vi "Disabled.vi"(7 "Robot Mode":T2, 10 "Match Info":T1={"Autonomous Elapsed Seconds"=0.0, "TeleOp Elapsed Seconds"=0.0, "Disabled Elapsed Seconds"=0.0, "Visited Autonomous"=FALSE, "Visited TeleOp"=FALSE, "Visited Disabled"=FALSE, "Autonomous Settings"={"Autonomous Style"=enum."Independent", "VI Refnum"=refnum}}, 11 "Call Context":T3) -> ()   [LabVIEW 2012]
doc: "This VI is called each time a disabled packet is received from the DS. It is often used to prepare for the next robot mode, to calibrate sensors, etc."
uses:
  <vilib>/Rock Robotics/WPI/DriverStation/WPI_DriverStationDerivedRobotMode.ctl
  <vilib>/Rock Robotics/WPI/DriverStation/WPI_DriverStationRobotMode2.ctl
  <vilib>/Rock Robotics/WPI/DriverStation/WPI_DriverStationMatch Info.ctl
  Robot Global Data.vi
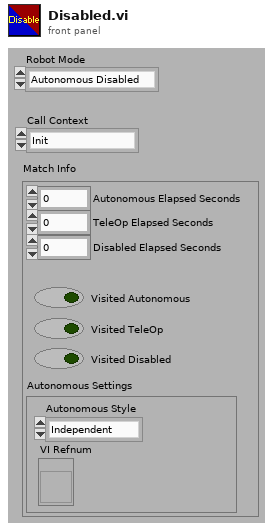
[diagram p1: front panel]
types:
  T1 = typedef "WPI_DriverStationMatch Info.ctl" = cluster{"Autonomous Elapsed Seconds":dbl, "TeleOp Elapsed Seconds":dbl, "Disabled Elapsed Seconds":dbl, "Visited Autonomous":bool, "Visited TeleOp":bool, "Visited Disabled":bool, "Autonomous Settings":cluster{"Autonomous Style":enum16{"Iterative", "Independent"}, "VI Refnum":refnum<vi>}}
  T2 = typedef "WPI_DriverStationRobotMode2.ctl" = enum16{"Autonomous Disabled", "Autonomous Enabled", "Teleop Disabled", "Teleop Enabled", "Timeout", "Finish", "Test Disabled", "Test Enabled"}
  T3 = typedef "WPI_DriverStationDerivedRobotMode.ctl" = enum16{"Init", "Execute", "Stop"}
  T4 = cluster{"FlipperLeftUp":dbl, "FlipperLeftDown":dbl, "FlipperRightUp":dbl, "FlipperRightDown":dbl, "KickerLeftBack":dbl, "KickerLeftForward":dbl, "KickerRightBack":dbl, "KickerRightForward":dbl}
  T5 = typedef "WPI_MotorControlDeviceRef.ctl" = cluster{"DeviceStatus":errorcluster, "Type":enum16{"PWM", "CAN"}, "PWM":cluster{"Digital Module":T6, "PWM Channel":T7, "DeadBand":T8}, "CAN":cluster{"Device Number":u8, "Control Mode":T9, "Semaphore":T10, "Max Vout":dbl}, "Invert":bool, "TransformRef":T11, "InvTransformRef":T11}
  T6 = typedef "FPGA_TypedefDigitalModule.ctl" = enum16{"Digital Module 1", "Digital Module 2"}
  T7 = typedef "FPGA_DIOPWMChannel.ctl" = enum8{"PWM 1", "PWM 2", "PWM 3", "PWM 4", "PWM 5", "PWM 6", "PWM 7", "PWM 8", "PWM 9", "PWM 10", "Invalid"}
  T8 = typedef "WPI_PWMDeadband.ctl" = cluster{"Name":string, "maxPositivePwm":i32, "minPositivePwm":i32, "centerPwm":i32, "maxNegativePwm":i32, "minNegativePwm":i32, "angularRange":u16}
  T9 = typedef "WPI_CANJaguar_ControlMode.ctl" = enum8{"Percent VBus", "Current", "Speed", "Position", "Voltage"}
  T10 = typedef "Semaphore RefNum" = refnum<k1>
  T11 = typedef "WPI_PWMTransform_ConPane.ctl" = refnum<vi>
  T12 = typedef "WPI_ServoDeviceRef.ctl" = cluster{"DeviceStatus":errorcluster, "Digital Module":T6, "PWM Channel":T7, "DeadBand":T8}
  T13 = cluster{"Right Servo High":dbl, "Right Servo Mid":dbl, "Right Servo Low":dbl, "Left Servo High":dbl, "Left Servo Mid":dbl, "Left Servo Low":dbl}
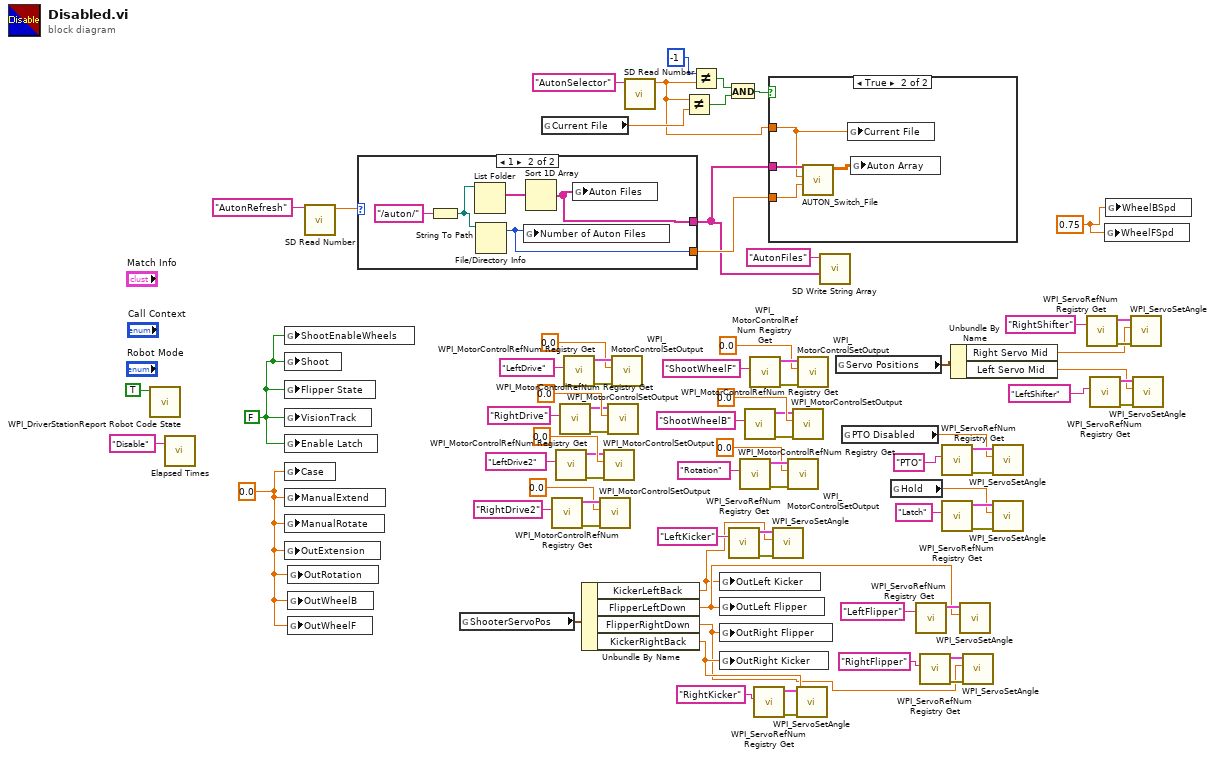
[diagram p0: block diagram]
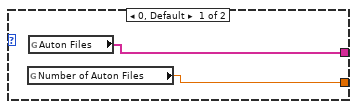
[diagram p3: hidden frame]
diagram:
  w1 = 0.75 ("Case")
  w24 = 0.0 ("Case")
  w25 = FALSE ("Enable Latch")
  n1 = call <vilib>:"WPI_DriverStationReport Robot Code State.vi"("Disabled"=TRUE ("Autonomous")) -> ()  [unwired: 10 in, 1 out]
  n2 = call "Elapsed Times.vi"("Call Name"="Disable") -> ()  [unwired: 2 in, 1 out]
  n3 = global write "Robot Global Data.vi" "ShootEnableWheels"(w25) -> ()
  n4 = global write "Robot Global Data.vi" "Shoot"(w25) -> ()
  n5 = global write "Robot Global Data.vi" "Flipper State"(w25) -> ()
  n6 = global write "Robot Global Data.vi" "VisionTrack"(w25) -> ()
  n7 = global write "Robot Global Data.vi" "Enable Latch"(w25) -> ()
  n8 = global write "Robot Global Data.vi" "Case"(w24) -> ()
  n9 = global write "Robot Global Data.vi" "ManualExtend"(w24) -> ()
  n10 = global write "Robot Global Data.vi" "ManualRotate"(w24) -> ()
  n11 = global write "Robot Global Data.vi" "OutExtension"(w24) -> ()
  n12 = global write "Robot Global Data.vi" "OutRotation"(w24) -> ()
  n13 = global write "Robot Global Data.vi" "OutWheelB"(w24) -> ()
  n14 = global write "Robot Global Data.vi" "OutWheelF"(w24) -> ()
  n15 = call <vilib>:"SD Read Number.vi"("Name"="AutonRefresh") -> ("Numeric"=w58:dbl)  [unwired: 8 in, 2 out]
  n16 = case shown="1" w58 {
    tunnel: [w79 w82] -> w68
    tunnel: [w80 w81] -> w63
    frame 0, Default {
      n17 = global read "Robot Global Data.vi" "Number of Auton Files"() -> (w79:dbl)
      n18 = global read "Robot Global Data.vi" "Auton Files"() -> (w80:string[])
    }
    frame 1 {
      n19 = String To Path(string="/auton/") -> (path=w84:path)
      n20 = List Folder(path=w84) -> (filenames=w83:string[])  [unwired: 3 in, 3 out]
      n21 = File/Directory Info(path=w84) -> (size=w82:i64)  [unwired: 1 in, 6 out]
      n22 = global write "Robot Global Data.vi" "Number of Auton Files"(w82) -> ()
      n23 = Sort 1D Array(array=w83) -> (sorted array=w81:string[])
      n24 = global write "Robot Global Data.vi" "Auton Files"(w81) -> ()
    }
  }
  n25 = global read "Robot Global Data.vi" "ShooterServoPos"() -> (w23:T4)
  n26 = global read "Robot Global Data.vi" "Current File"() -> (w66:dbl)
  n27 = call <vilib>:"WPI_MotorControlRefNum Registry Get.vi"("refnum name"="RightDrive2") -> ("error out"=w44:errorcluster, "MotorControlDevRef"=w43:T5)  [unwired: 9 in]
  n28 = call <vilib>:"WPI_MotorControlRefNum Registry Get.vi"("refnum name"="LeftDrive2") -> ("error out"=w37:errorcluster, "MotorControlDevRef"=w38:T5)  [unwired: 9 in]
  n29 = call <vilib>:"WPI_MotorControlRefNum Registry Get.vi"("refnum name"="RightDrive") -> ("error out"=w69:errorcluster, "MotorControlDevRef"=w70:T5)  [unwired: 9 in]
  n30 = call <vilib>:"WPI_MotorControlRefNum Registry Get.vi"("refnum name"="LeftDrive") -> ("error out"=w76:errorcluster, "MotorControlDevRef"=w75:T5)  [unwired: 9 in]
  n31 = Unbundle By Name(w23) -> ("KickerLeftBack"=w20:dbl, "FlipperLeftDown"=w21:dbl, "FlipperRightDown"=w19:dbl, "KickerRightBack"=w22:dbl)
  n32 = call <vilib>:"WPI_MotorControlSetOutput.vi"("error in (no error)"=w44, "Output"=0.0, "MotorControlDevRef"=w43) -> ()  [unwired: 6 in, 3 out]
  n33 = call <vilib>:"WPI_MotorControlSetOutput.vi"("error in (no error)"=w37, "Output"=0.0, "MotorControlDevRef"=w38) -> ()  [unwired: 6 in, 3 out]
  n34 = call <vilib>:"WPI_MotorControlSetOutput.vi"("error in (no error)"=w69, "Output"=0.0, "MotorControlDevRef"=w70) -> ()  [unwired: 6 in, 3 out]
  n35 = call <vilib>:"WPI_MotorControlSetOutput.vi"("error in (no error)"=w76, "Output"=0.0, "MotorControlDevRef"=w75) -> ()  [unwired: 6 in, 3 out]
  n36 = call <vilib>:"SD Read Number.vi"("Name"="AutonSelector") -> ("Numeric"=w59:dbl)  [unwired: 8 in, 2 out]
  n37 = Not Equal?(x=w59, y=w66) -> (x != y?=w64:bool)
  n38 = Not Equal?(x=-1, y=w59) -> (x != y?=w65:bool)
  n39 = global write "Robot Global Data.vi" "OutLeft Kicker"(w20) -> ()
  n40 = global write "Robot Global Data.vi" "OutLeft Flipper"(w21) -> ()
  n41 = global write "Robot Global Data.vi" "OutRight Flipper"(w19) -> ()
  n42 = global write "Robot Global Data.vi" "OutRight Kicker"(w22) -> ()
  n43 = And(x=w65, y=w64) -> (x .and. y?=w61:bool)
  n44 = call <vilib>:"WPI_ServoRefNum Registry Get.vi"("refnum name"="LeftKicker") -> ("error out"=w26:errorcluster, "ServoDeviceRef"=w27:T12)  [unwired: 9 in]
  n45 = call <vilib>:"WPI_MotorControlRefNum Registry Get.vi"("refnum name"="Rotation") -> ("error out"=w48:errorcluster, "MotorControlDevRef"=w47:T5)  [unwired: 9 in]
  n46 = call <vilib>:"WPI_MotorControlRefNum Registry Get.vi"("refnum name"="ShootWheelB") -> ("error out"=w49:errorcluster, "MotorControlDevRef"=w50:T5)  [unwired: 9 in]
  n47 = call <vilib>:"WPI_MotorControlRefNum Registry Get.vi"("refnum name"="ShootWheelF") -> ("error out"=w56:errorcluster, "MotorControlDevRef"=w55:T5)  [unwired: 9 in]
  n48 = call <vilib>:"WPI_ServoRefNum Registry Get.vi"("refnum name"="RightKicker") -> ("error out"=w34:errorcluster, "ServoDeviceRef"=w32:T12)  [unwired: 9 in]
  n49 = case shown="True" w61 {
    tunnel: w63 -> [_ w89]
    tunnel: w68 -> [_ w88]
    tunnel: w59 -> [_ w86]
    frame False {
    }
    frame True {
      n50 = call "AUTON_Switch_File.vi"("Number of Auton Files"=w88, "Auton File"=w86, "Auton Files"=w89) -> ("Auton Array"=w87:dbl[][])  [unwired: 7 in, 1 out]
      n51 = global write "Robot Global Data.vi" "Current File"(w86) -> ()
      n52 = global write "Robot Global Data.vi" "Auton Array"(w87) -> ()
    }
  }
  n53 = call <vilib>:"WPI_ServoSetAngle.vi"("error in (no error)"=w26, "Angle"=w20, "ServoDeviceRef"=w27) -> ()  [unwired: 7 in, 2 out]
  n54 = call <vilib>:"WPI_MotorControlSetOutput.vi"("error in (no error)"=w48, "Output"=0.0, "MotorControlDevRef"=w47) -> ()  [unwired: 6 in, 3 out]
  n55 = call <vilib>:"WPI_MotorControlSetOutput.vi"("error in (no error)"=w49, "Output"=0.0, "MotorControlDevRef"=w50) -> ()  [unwired: 6 in, 3 out]
  n56 = call <vilib>:"WPI_ServoSetAngle.vi"("error in (no error)"=w34, "Angle"=w22, "ServoDeviceRef"=w32) -> ()  [unwired: 7 in, 2 out]
  n57 = call <vilib>:"WPI_MotorControlSetOutput.vi"("error in (no error)"=w56, "Output"=0.0, "MotorControlDevRef"=w55) -> ()  [unwired: 6 in, 3 out]
  n58 = call <vilib>:"SD Write String Array.vi"("String Array"=w63, "Name"="AutonFiles") -> ()  [unwired: 8 in, 2 out]
  n59 = global read "Robot Global Data.vi" "Servo Positions"() -> (w6:T13)
  n60 = global read "Robot Global Data.vi" "PTO Disabled"() -> (w3:dbl)
  n61 = global read "Robot Global Data.vi" "Hold"() -> (w2:dbl)
  n62 = call <vilib>:"WPI_ServoRefNum Registry Get.vi"("refnum name"="LeftFlipper") -> ("ServoDeviceRef"=w28:T12)  [unwired: 9 in, 1 out]
  n63 = call <vilib>:"WPI_ServoRefNum Registry Get.vi"("refnum name"="RightFlipper") -> ("error out"=w36:errorcluster, "ServoDeviceRef"=w29:T12)  [unwired: 9 in]
  n64 = call <vilib>:"WPI_ServoRefNum Registry Get.vi"("refnum name"="PTO") -> ("error out"=w9:errorcluster, "ServoDeviceRef"=w12:T12)  [unwired: 9 in]
  n65 = call <vilib>:"WPI_ServoRefNum Registry Get.vi"("refnum name"="Latch") -> ("error out"=w7:errorcluster, "ServoDeviceRef"=w8:T12)  [unwired: 9 in]
  n66 = Unbundle By Name(w6) -> ("Right Servo Mid"=w4:dbl, "Left Servo Mid"=w5:dbl)
  n67 = call <vilib>:"WPI_ServoSetAngle.vi"("Angle"=w21, "ServoDeviceRef"=w28) -> ()  [unwired: 8 in, 2 out]
  n68 = call <vilib>:"WPI_ServoSetAngle.vi"("error in (no error)"=w36, "Angle"=w19, "ServoDeviceRef"=w29) -> ()  [unwired: 7 in, 2 out]
  n69 = call <vilib>:"WPI_ServoSetAngle.vi"("error in (no error)"=w9, "Angle"=w3, "ServoDeviceRef"=w12) -> ()  [unwired: 7 in, 2 out]
  n70 = call <vilib>:"WPI_ServoSetAngle.vi"("error in (no error)"=w7, "Angle"=w2, "ServoDeviceRef"=w8) -> ()  [unwired: 7 in, 2 out]
  n71 = call <vilib>:"WPI_ServoRefNum Registry Get.vi"("refnum name"="RightShifter") -> ("error out"=w15:errorcluster, "ServoDeviceRef"=w16:T12)  [unwired: 9 in]
  n72 = call <vilib>:"WPI_ServoRefNum Registry Get.vi"("refnum name"="LeftShifter") -> ("error out"=w17:errorcluster, "ServoDeviceRef"=w18:T12)  [unwired: 9 in]
  n73 = global write "Robot Global Data.vi" "WheelFSpd"(w1) -> ()
  n74 = global write "Robot Global Data.vi" "WheelBSpd"(w1) -> ()
  n75 = call <vilib>:"WPI_ServoSetAngle.vi"("error in (no error)"=w15, "Angle"=w4, "ServoDeviceRef"=w16) -> ()  [unwired: 7 in, 2 out]
  n76 = call <vilib>:"WPI_ServoSetAngle.vi"("error in (no error)"=w17, "Angle"=w5, "ServoDeviceRef"=w18) -> ()  [unwired: 7 in, 2 out]
